vi "Search for Valid Port.vi"() -> (1 "Version":string, 2 "CAT Port?":bool, 3 "Port Out":refnum<visa-resource-name>)   [LabVIEW 2013]
doc: "When a connection has been dropped - i.e. the port we were connected to is no longer valid - the system may have to hunt for a new connection. This is because, in the most catastrophic case, the port on which the device had been previously connected is not the new port that the device will be talking on. This might happen if the user removed a USB to serial converter and then plugged the converter back into a different USB port if a different cable was plugged in.\n\nIn order to find the correct port, the system first calls the VISA Find Resources to determine what connections are available. This VI then loops through the list, configuring, opening and then polling the port with the request for the CAT Engine version. If the device on the port responds (i.e. the number of bytes is not zero), then the VI returns TRUE on the indicator <b>CAT Port?</b> and the correct resource on <b>Port Out</b>."
uses:
  <vilib>/Instr/_visa.llb/VISA Find Search Mode.ctl
  Type Defs/Comm Settings.ctl
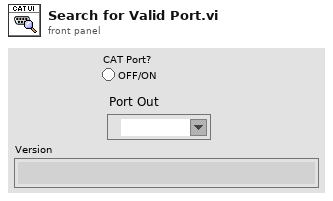
[diagram p1: front panel]
types:
  T1 = typedef "Comm Settings.ctl" = cluster{"Port":refnum<visa-resource-name>, "Baud Rate":u32, "Data Bits":u16, "Parity":u16, "Stop Bits":u16, "Flow Control":u16}
  T2 = typedef "VISA Find Search Mode.ctl" = u32
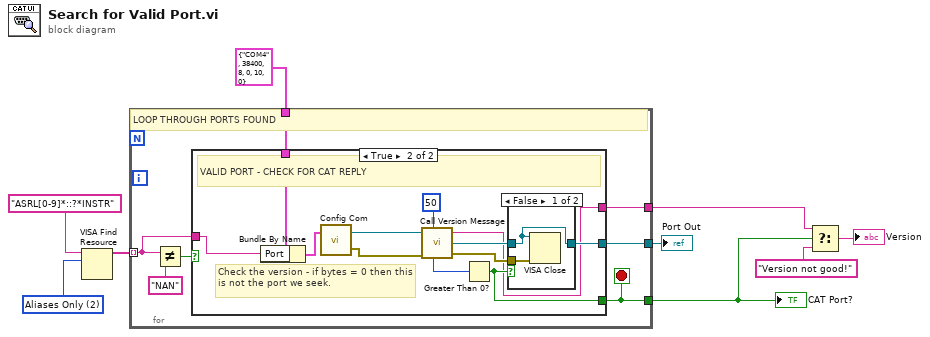
[diagram p0: block diagram]
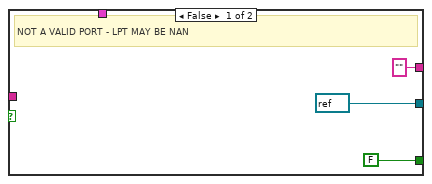
[diagram p2: hidden frame]
diagram:
  w9 = T2 2 items=["Canonical Names Only"=0, "Aliases Only"=2, "Include Matching Aliases"=3, "Include All Aliases"=4] ("Search Mode")
  n1 = VISA Find Resource(10:w9, 11:"ASRL[0-9]*::?*INSTR" ("expression (\"?*\")")) -> (3:w7:string[])  [unwired: 1 in, 2 out]
  n2 = for {
    tunnel: w7 -> [w14] mode=indexing
    tunnel: [w13] -> w4
    tunnel: T1 {"Port"="COM4", "Baud Rate"=38400, "Data Bits"=8, "Parity"=0, "Stop Bits"=10, "Flow Control"=0} ("Com Parms") -> [w12]
    tunnel: [w11] -> w5
    tunnel: [w10] -> w3
    stop <- w13 stop-if-true
    # "LOOP THROUGH PORTS FOUND"
    n3 = Not Equal?(x=w14, y="NAN" ("x")) -> (x != y?=w15:bool)
    n4 = case shown="True" w15 {
      tunnel: w14 -> [_ w24]
      tunnel: [FALSE w29] -> w13
      tunnel: w12 -> [_ w25]
      tunnel: [refnum<visa-resource-name> refnum ("VISA resource name out 2") w26] -> w11
      tunnel: ["" ("read string") w20] -> w10
      frame False {
        # "NOT A VALID PORT - LPT MAY BE NAN"
      }
      frame True {
        # "Check the version - if bytes = 0 then this is not the port we seek."
        # "VALID PORT - CHECK FOR CAT REPLY"
        n5 = Bundle By Name(cluster=w25, "Port"=w24) -> (w23:T1)
        n6 = call "Config Com.vi"("Com Parms"=w23) -> ("error out"=w22:errorcluster, "VISA resource name out"=w21:refnum<visa-resource-name>)  [unwired: 1 in]
        n7 = call "Call Version Message.vi"("VISA resource name out"=w21, "delay before read (ms)"=u32 50, "error in"=w22) -> ("bytes read"=w30:u32, "read string"=w20:string, "VISA Out"=w28:refnum<visa-resource-name>, "error out"=w27:errorcluster)  [unwired: 2 in]
        n8 = Greater Than 0?(x=w30) -> (x > 0?=w29:bool)
        n9 = case shown="False" w29 {
          tunnel: w28 -> [w32 w34]
          tunnel: w27 -> [w33 _]
          tunnel: [w32 w34] -> w26
          frame False {
            n10 = VISA Close(VISA resource name=w32, error in (no error)=w33) -> ()  [unwired: 1 out]
          }
          frame True {
          }
        }
      }
    }
  }
  "CAT Port?" <- w4
  "Port Out" <- w5
  n11 = Select(t=w3, s=w4, f="Version not good!") -> (s? t:f=→"Version":string)
